vi "DiffKinematics_toWheelSpeed.vi"(9 "TrackWidth_Meters":dbl, 11 "CHASSIS Speed":T1) -> (1 "RightVelocity":dbl, 3 "LeftVelocity":dbl)   [LabVIEW 2019, in "PathExecution_Library.lvlib"]
uses:
  PathExecution_Library.lvlib
  CHASSIS.ctl
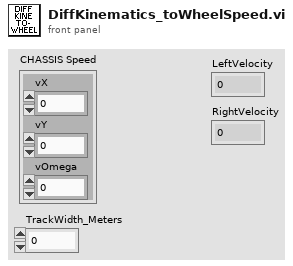
[diagram p1: front panel]
types:
  T1 = typedef "PathExecution_Library.lvlib/CHASSIS.ctl" = cluster{"vX":dbl, "vY":dbl, "vOmega":dbl}
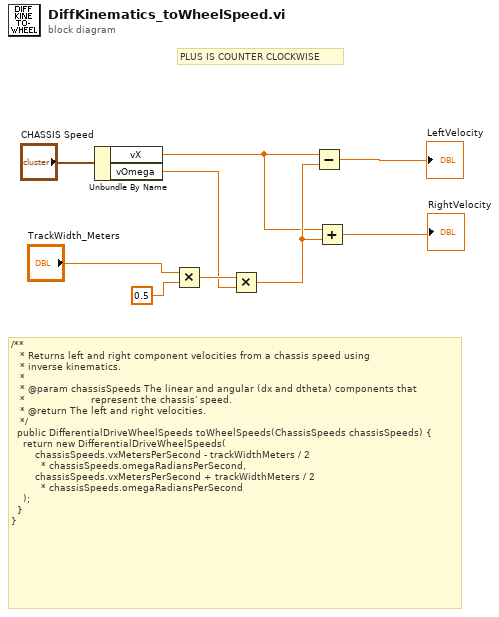
[diagram p0: block diagram]
diagram:
  # "PLUS IS COUNTER CLOCKWISE"
  # "/**\n   * Returns left and right component velocities from a chassis speed using\n   * inverse kinematics.\n   *\n   * @param chassisSpeeds The linear and angular (dx and dtheta) components that\n   *                      represent the chassis' speed.\n   * @return The left and right velocities.\n   */\n  public DifferentialDriveWheelSpeeds toWheelSpeeds(ChassisSpeeds chassisSpeeds) {\n    return new DifferentialDriveWheelSpeeds(\n        chassisSpeeds.vxMetersPerSecond - trackWidthMeters / 2\n          * chassisSpeeds.omegaRadiansPerSecond,\n        chassisSpeeds.vxMetersPerSecond + trackWidthMeters / 2\n          * chassisSpeeds.omegaRadiansPerSecond\n    );\n  }\n}"
  n1 = Unbundle By Name("CHASSIS Speed") -> ("vX"=w2:dbl, "vOmega"=w1:dbl)
  n2 = Multiply(x="TrackWidth_Meters", y=0.5) -> (x*y=w7:dbl)
  n3 = Multiply(x=w7, y=w1) -> (x*y=w6:dbl)
  n4 = Subtract(x=w2, y=w6) -> (x-y=→"LeftVelocity":dbl)
  n5 = Add(x=w2, y=w6) -> (x+y=→"RightVelocity":dbl)
